vi "Capture Millisecond Tick Elapsed Time.vi"(6 "bypass Q (F)":bool, 7 "comment":string, 8 "error in (no error)":errorcluster, 10 "idx (0)":i32, 11 "DbgTimers in":refnum<class "DbgTimers.lvclass">) -> (0 "error out":errorcluster, 1 "timed out?":bool, 3 "DbgTimers out":refnum<class "DbgTimers.lvclass">)   [LabVIEW 2017, in "DbgTimers.lvclass"]
doc: "Developed by Kevin Thompson\nkevin@thompsonengineering.net\n\nCopyright 2018-2020\nThompson Engineering, LLC"
uses:
  DbgTimers.lvclass
  DataTypes/Millsecond Tick Timer Qdata--cluster.ctl
  DataTypes/Millisecond Tick Timer--cluster.ctl
  DbgTimers.lvclass/DbgTimers.ctl
  Accessors/Get ObjData.vi
  Accessors/Set ObjData.vi
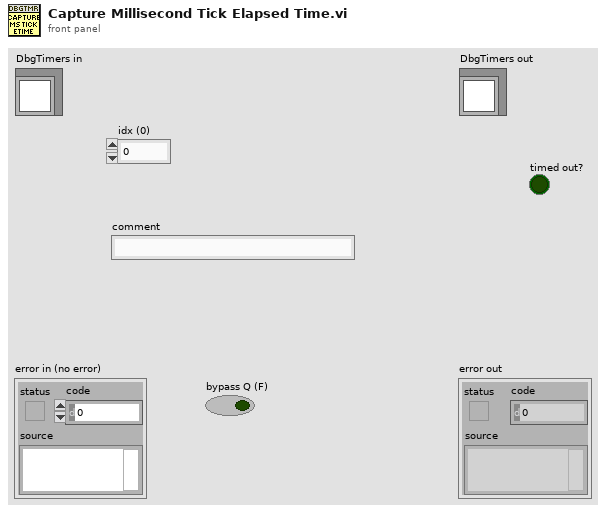
[diagram p1: front panel]
types:
  T1 = typedef "DbgTimers.lvclass/Millsecond Tick Timer Qdata--cluster.ctl" = cluster{"Time Stamp":timestamp, "comment":string, "idx":i32, "ms tick timer":T2}
  T2 = typedef "DbgTimers.lvclass/Millisecond Tick Timer--cluster.ctl" = cluster{"startTick":u32, "currentTick":u32, "elapsedTicks":u32, "totalElapsedTicks":u32}
  T3 = typedef "DbgTimers.lvclass/ObjData--cluster.ctl" = cluster{"Settings":T4, "ReadData-placeholder":T5, "Timers":T6, "Enable msTick Logging":bool, "LogFile_msTickTimer":path}
  T4 = typedef "DbgTimers.lvclass/Settings--cluster.ctl" = cluster{"Simulation":bool, "DbgTimer LogFolder":path}
  T5 = typedef "DbgTimers.lvclass/Read Data--cluster.ctl" = cluster{"Data":dbl}
  T6 = typedef "DbgTimers.lvclass/Timers--cluster.ctl" = cluster{"ms tick timers":T2[]}
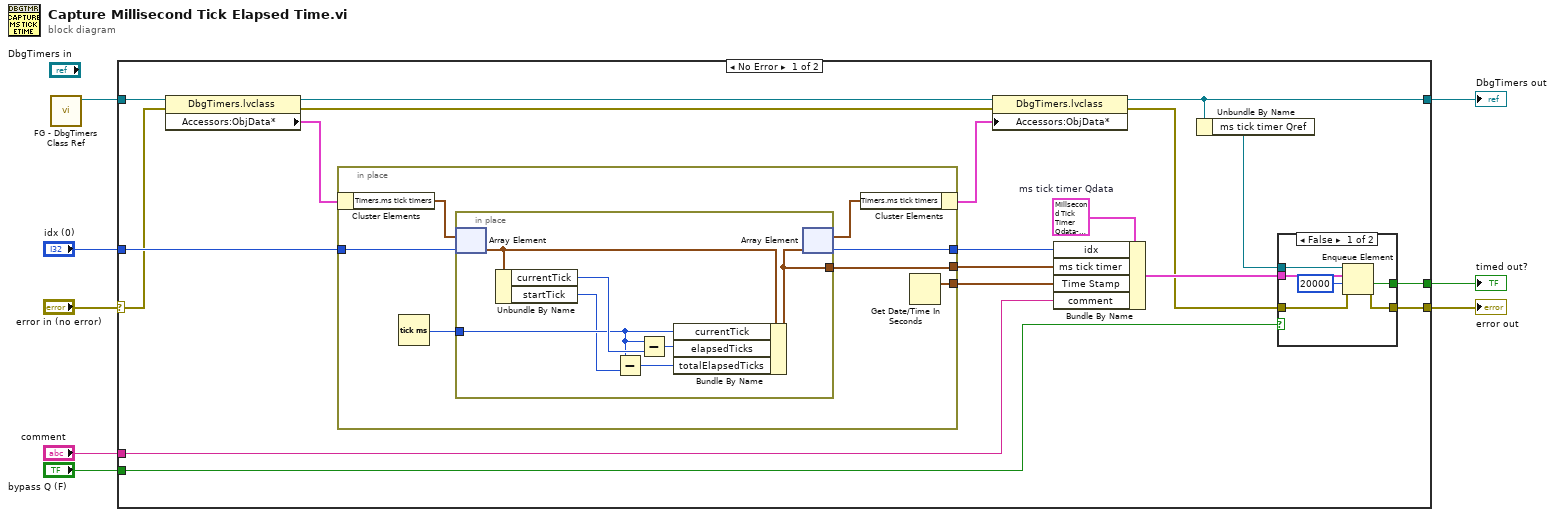
[diagram p0: block diagram]
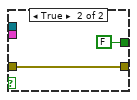
[diagram p2: hidden frame]
diagram:
  n1 = call "FG - DbgTimers Class Ref.vi"() -> ("DbgTimers out"=w1:refnum<class "DbgTimers.lvclass">)  [unwired: 9 in, 1 out]
  n2 = case shown="No Error" "error in (no error)" {
    selector: "error in (no error)" -> [w18 w51]
    tunnel: [w9 w51] -> w7
    tunnel: [w16 w50] -> w6
    tunnel: w1 -> [w27 w50]
    tunnel: "idx (0)" -> [w24 _]
    tunnel: "comment" -> [w20 _]
    tunnel: [w14 _] -> w3
    tunnel: "bypass Q (F)" -> [w13 _]
    frame No Error {
      w22 = T1 {"Time Stamp"=timestamp(0 s since 1904-01-01), "comment"="", "idx"=0, "ms tick timer"={"startTick"=0, "currentTick"=0, "elapsedTicks"=0, "totalElapsedTicks"=0}}  # ms tick timer Qdata
      n3 = property class="DbgTimers.lvclass"(reference=w27, error in=w18) -> (reference out=w26:refnum<class "DbgTimers.lvclass">, error out=w23:errorcluster, "Accessors:ObjData*"=w25:T3)
      n4 = in-place {
        in-place-border: w24 -> [w42]
        in-place-border: [w39] -> w21
        in-place-border: [w37] -> w12
        in-place-border: [w36] -> w11
        n5 = in-place-cluster #1(w25) -> ("Timers.ms tick timers"=w41:T2[])
        n6 = Tick Count (ms)() -> (millisecond timer value=w38:u32)
        n7 = in-place {
          in-place-border: w38 -> [w45]
          in-place-border: [w49] -> w39
          n8 = in-place-array #2(w41, w42) -> (w48:T2)
          n9 = Unbundle By Name(w48) -> ("currentTick"=w46:u32, "startTick"=w44:u32)
          n10 = Subtract(x=w45, y=w44) -> (x-y=w43:u32)
          n11 = Subtract(x=w45, y=w46) -> (x-y=w47:u32)
          n12 = Bundle By Name(cluster=w48, "currentTick"=w45, "elapsedTicks"=w47, "totalElapsedTicks"=w43) -> (w49:T2)
          n13 = in-place-array #2(w49) -> (w40:T2[], w37:i32)
        }
        n14 = in-place-cluster #1("Timers.ms tick timers"=w40) -> (w17:T3)
        n15 = Get Date/Time In Seconds() -> (seconds since 1Jan1904=w36:timestamp)
      }
      n16 = property class="DbgTimers.lvclass"(reference=w26, error in=w23, "Accessors:ObjData*"=w17) -> (reference out=w16:refnum<class "DbgTimers.lvclass">, error out=w10:errorcluster)
      n17 = Bundle By Name(cluster=w22, "idx"=w12, "ms tick timer"=w21, "Time Stamp"=w11, "comment"=w20) -> (w19:T1)
      n18 = Unbundle By Name(w16) -> ("ms tick timer Qref"=w15:refnum<queue>)
      n19 = case shown="False" w13 {
        tunnel: w19 -> [w33 _]
        tunnel: w15 -> [w32 _]
        tunnel: [w30 FALSE ("timed out?")] -> w14
        tunnel: w10 -> [w29 w35]
        tunnel: [w28 w35] -> w9
        frame False {
          n20 = Enqueue Element(queue=w32, element=w33, timeout in ms (-1)=20000, error in (no error)=w29) -> (timed out?=w30:bool, error out=w28:errorcluster)  [unwired: 1 out]
        }
        frame True {
        }
      }
    }
    frame Error {
    }
  }
  "error out" <- w7
  "DbgTimers out" <- w6
  "timed out?" <- w3
